vi "SCMP FITS Writer.vi"(5 "Andor":T1={"Handle"=0, "Pixel Encoding"="", "AOI Width"=0, "AOI Height"=0, "AOI Stride"=0, "Row Readout Time"=0.0, "Frame Readout Time"=0.0, "Interframe Time"=0.0, "Semaphore"=refnum, "SerialNumber"="", "Camera Model"="", "Controller ID"="", "Firmware Version"="", "Shutter"="Global", "BDiv"=1, "Time at Synch"=timestamp(3029526000.379448 s since 1904-01-01), "Idx"=0, "PreAmp"="", "Binning"=enum."1x1", "PixelReadoutRate"="", "Exposure (s)"=0.05, "Image Bytes"=0, "Image Pixels"=0, "SpuriousNoiseFilter"=FALSE, "Overlap"=FALSE, "CycleMode"=""} {"Exposure (s)" format="%^.3g"; "Time at Synch" format="%<%H:%M:%S>T"; "Interframe Time" format="%#_3g"; "Frame Readout Time" format="%_3g"; "Row Readout Time" format="%_3g"}, 7 "FITS Cluster":T4={"Wavelength (nm)"=530.15, "Exposure (s)"=0.05, "Tuning Delay (ms)"=1000.0, "Beam Type (-1/1)"=1.0, "Tuning Voltages"=[1.111, 2.222, 3.333, 4.444], "Observer"="observer", "Light Shapping Diffuser"=enum."In Beam", "Comment"="", "Data Type"=9, "Mod Cycles"=0, "SCD Calibration Optics"=enum."1 - Polarizer @0, I+Q", "SCD Emission Line Filter"=enum."1-557.6nm", "Cookbook"="", "COMP-S Calibration Wheel"=enum."Dark", "COMP-S Andover Filter Wheel"=enum."530.3nm/HWB 0.34nm (Fe XIV)", "FOV Rotation (deg)"=66.0, "Objective Lens Position (mm)"=0.0, "Occulter size"=0.0, "Time End"=timestamp(3382374145.421875 s since 1904-01-01), "Acc Exposure (s)"=0.0, "Time Stamp Array"=[], "Camera Serial Number"=[], "Camera Temp"=[], "Camera PI (mm)"=[], "Time Start"=timestamp(3382374145.421875 s since 1904-01-01), "Peripherals"={"ILX controler"=FALSE, "Zone temperatures"=FALSE, "Andor"=FALSE, "Andor 2"=FALSE, "PI Stages"=FALSE, "AISAS mechanisms"=FALSE, "AISAS Mech.lvclass"=refnum, "Zone temp ref"=variant, "FWs"=FALSE}, "FITS paths"=[], "Cameras"=enum."Andor", "load preset cbk"=FALSE, "periodic check count"=0} {"Camera PI (mm)" format="%_3g"; "Acc Exposure (s)" format="%^.3g"; "Occulter size" format="%.2f"; "Objective Lens Position (mm)" min=70.0 max=152.0 format="%.2f"; "FOV Rotation (deg)" format="%.1f"; "Data Type" items=["LIVE", "DARK", "FLAT", "CALI", "OBSE", "ABSO", "AURE", "TARG", "OBJE", "HOLE", "OREX", "THRO", "CHIP"]; "Exposure (s)" format="%^.3g"; "Wavelength (nm)" format="%_6g"}, 8 "error in":errorcluster, 10 "Image Vector":u32[](array[numeric]), 11 "Wavelength (0..n)":i32) -> (0 "error out":errorcluster, 3 "Current FITS Path":path)   [LabVIEW 2014]
doc: "Use this template to build a VI to use as a subVI."
uses:
  Controls/SCD - FITS Cluster.ctl
  AISAS/Mech/AISAS Mech.lvclass
  AISAS/Controls/Diffuser.ctl
  Controls/SCD - Calibration Optics Filter Wheel.ctl
  Controls/SCD - EDT - Emission Line Filter Wheel.ctl
  Controls/CoMP-S Controls/Polarization Optics Filter Wheel.ctl
  Controls/CoMP-S Controls/Emission Line Filter Wheel.ctl
  AISAS/Controls/focus.ctl
  Controls/peripherals.ctl
  Controls/Cameras select.ctl
  Camera/Andor Neo Info.ctl
  Controls/beaning.ctl
panel:
  out "FITS Path static":path=path "G:/SCD Data/Level-0/20160930/20160930T203514.fits"
  out "1st Extension Header":string="XTENSION=                        'IMAGE' /                                      BITPIX  =                             32 / BITS PER PIXEL                       NAXIS   =                              3 / NUMBER OF AXES (2)                   NAXIS1  =                           2560 / XDIM (PIXELS)                        NAXIS2  =                           2160 / YDIM (PIXELS)                        NAXIS3  =                              4 / 4 POLARIZATION STATES                GCOUNT  =                              1 /                                      TIME_OBS=                   '203202.348' / TIME OF OBSERVATION (UTC)            DATE_END=                                / DATE OF OBSERVATION END (UTC)        EXPOSURE=                       0.020000 / EXPOSURE TIME (MILLISEC)             PCOUNT  =                              0 /                                      BZERO   =                             0. / 32768.                               BSCALE  =                             1. / 1                                    MODC    =                              3 / NUMBER OF IMAGES AT EACH STATE       WAVELENG=                         656.20 / WAVELENGTH OF OBS (NM)               COMMENT                                                                         COMMENT                                                                         COMMENT                                                                         COMMENT                                                                         COMMENT                                                                         COMMENT                                                                         COMMENT                                                                         COMMENT                                                                         COMMENT                                                                         COMMENT                                                                         COMMENT                                                                         COMMENT                                                                         COMMENT                                                                         COMMENT                                                                         COMMENT                                                                         COMMENT                                                                         COMMENT                                                                         COMMENT                                                                         COMMENT                                                                         COMMENT                                                                         COMMENT                                                                         COMMENT                                                                         COMMENT                                                                         COMMENT                                                                         COMMENT                                                                         COMMENT                                                                         COMMENT                                                                         COMMENT                                                                         COMMENT                                                                         COMMENT                                                                         COMMENT                                                                         COMMENT                                                                         COMMENT                                                                         COMMENT                                                                         COMMENT                                                                         COMMENT                                                                         COMMENT                                                                         COMMENT                                                                         COMMENT                                                                         COMMENT                                                                         COMMENT                                                                         COMMENT                                                                         COMMENT                                                                         COMMENT                                                                         COMMENT                                                                         COMMENT                                                                         COMMENT                                                                         COMMENT                                                                         COMMENT                                                                         COMMENT                                                                         COMMENT                                                                         COMMENT                                                                         COMMENT                                                                         COMMENT                                                                         COMMENT                                                                         COMMENT                                                                         COMMENT                                                                         COMMENT                                                                         COMMENT                                                                         COMMENT                                                                         COMMENT                                                                         COMMENT                                                                         COMMENT                                                                         COMMENT                                                                         COMMENT                                                                         COMMENT                                                                         COMMENT                                                                         COMMENT                                                                         COMMENT                                                                         COMMENT                                                                         COMMENT                                                                         COMMENT                                                                         COMMENT                                                                         COMMENT                                                                         COMMENT                                                                         COMMENT                                                                         COMMENT                                                                         COMMENT                                                                         COMMENT                                                                         COMMENT                                                                         COMMENT                                                                         COMMENT                                                                         COMMENT                                                                         COMMENT                                                                         COMMENT                                                                         COMMENT                                                                         COMMENT                                                                         COMMENT                                                                         COMMENT                                                                         COMMENT                                                                         COMMENT                                                                         COMMENT                                                                         COMMENT                                                                         COMMENT                                                                         COMMENT                                                                         COMMENT                                                                         COMMENT                                                                         COMMENT                                                                         COMMENT                                                                         COMMENT                                                                         COMMENT                                                                         COMMENT                                                                         COMMENT                                                                         COMMENT                                                                         COMMENT                                                                         COMMENT                                                                         COMMENT                                                                         COMMENT                                                                         COMMENT                                                                         COMMENT                                                                         COMMENT                                                                         COMMENT                                                                         COMMENT                                                                         COMMENT                                                                         COMMENT                                                                         COMMENT                                                                         COMMENT                                                                         COMMENT                                                                         COMMENT                                                                         COMMENT                                                                         COMMENT                                                                         COMMENT                                                                         COMMENT                                                                         COMMENT                                                                         COMMENT                                                                         COMMENT                                                                         COMMENT                                                                         COMMENT                                                                         COMMENT                                                                         COMMENT                                                                         COMMENT                                                                         COMMENT                                                                         COMMENT                                                                         COMMENT                                                                         COMMENT                                                                         COMMENT                                                                         COMMENT                                                                         COMMENT                                                                         COMMENT                                                                         COMMENT                                                                         COMMENT                                                                         COMMENT                                                                         COMMENT                                                                         COMMENT                                                                         COMMENT                                                                         COMMENT                                                                         COMMENT                                                                         COMMENT                                                                         COMMENT                                                                         COMMENT                                                                         COMMENT                                                                         COMMENT                                                                         COMMENT                                                                         COMMENT                                                                         COMMENT                                                                         COMMENT                                                                         COMMENT                                                                         COMMENT                                                                         COMMENT                                                                         COMMENT                                                                         COMMENT                                                                         COMMENT                                                                         COMMENT                                                                         COMMENT                                                                         COMMENT                                                                         COMMENT                                                                         COMMENT                                                                         COMMENT                                                                         COMMENT                                                                         COMMENT                                                                         COMMENT                                                                         COMMENT                                                                         COMMENT                                                                         COMMENT                                                                         COMMENT                                                                         COMMENT                                                                         COMMENT                                                                         COMMENT                                                                         COMMENT                                                                         COMMENT                                                                         COMMENT                                                                         COMMENT                                                                         COMMENT                                                                         COMMENT                                                                         COMMENT                                                                         COMMENT                                                                         COMMENT                                                                         COMMENT                                                                         COMMENT                                                                         COMMENT                                                                         COMMENT                                                                         COMMENT                                                                         COMMENT                                                                         COMMENT                                                                         COMMENT                                                                         COMMENT                                                                         COMMENT                                                                         COMMENT                                                                         COMMENT                                                                         COMMENT                                                                         COMMENT                                                                         COMMENT                                                                         COMMENT                                                                         COMMENT                                                                         COMMENT                                                                         COMMENT                                                                         COMMENT                                                                         COMMENT                                                                         COMMENT                                                                         COMMENT                                                                         COMMENT                                                                         COMMENT                                                                         COMMENT                                                                         COMMENT                                                                         COMMENT                                                                         COMMENT                                                                         COMMENT                                                                         COMMENT                                                                         COMMENT                                                                         COMMENT                                                                         COMMENT                                                                         COMMENT                                                                         COMMENT                                                                         COMMENT                                                                         COMMENT                                                                         COMMENT                                                                         COMMENT                                                                         COMMENT                                                                         COMMENT                                                                         COMMENT                                                                         COMMENT                                                                         COMMENT                                                                         COMMENT                                                                         COMMENT                                                                         COMMENT                                                                         COMMENT                                                                         COMMENT                                                                         COMMENT                                                                         COMMENT                                                                         COMMENT                                                                         COMMENT                                                                         COMMENT                                                                         COMMENT                                                                         COMMENT                                                                         COMMENT                                                                         COMMENT                                                                         COMMENT                                                                         COMMENT                                                                         COMMENT                                                                         COMMENT                                                                         COMMENT                                                                         COMMENT                                                                         COMMENT                                                                         COMMENT                                                                         COMMENT                                                                         COMMENT                                                                         COMMENT                                                                         COMMENT                                                                         COMMENT                                                                         COMMENT                                                                         COMMENT                                                                         COMMENT                                                                         COMMENT                                                                         COMMENT                                                                         COMMENT                                                                         COMMENT                                                                         COMMENT                                                                         COMMENT                                                                         COMMENT                                                                         COMMENT                                                                         COMMENT                                                                         COMMENT                                                                         END                                                                             "
  out "Primary Header":string="SIMPLE  =                              T / CONFORMS TO FITS STANDARD            BITPIX  =                             32 / BITS PER PIXEL                       NAXIS   =                              0 / DATA DIMENSIONS IN FITS FILE         NAXIS1  =                           2560 / XDIM (PIXELS)                        NAXIS2  =                           2160 / YDIM (PIXELS)                        NAXIS3  =                              4 / 4 POLARIZATION STATES                NAXIS4  =                              1 / 1 CAMERA                             EXTEND  =                              T / EXTENSIONS POSSIBLE                  OBSERVER=                       'Sewell' / NAME OF OBSERVER                     TELESCOP=                   '20CM ZEISS' / NAME OF TELESCOPE                    LOCATION=            'LOMNICKY PEAK OBS' / LOCATION OF TELESCOPE                INSTRUME=                          'SCD' / NAME OF INSTRUMENT                   BZERO   =                             0. /  ADU OFFSET                          FOCUS   =                     -22.000000 / CAMERA-STAGE POSITION (MM)           ROTPOS  =                            0.0 / ROTATIONAL POSITION (DEG)            DIFFUSER=                      'IN BEAM' / 0=IN BEAM, 1=OUT OF BEAM             FW-WVLNG=                        '656.4' / PRE-FILTER CENTER WAVELENGTH (NM)    FW-CALIB=                         'Dark' / CAL-WHEEL POSITION                   CAM-SN1 =                    'SCC-02209' / CAMERA SERIAL NUMBER                 CAM-TEMP=                     -19.610000 / FOCAL PLANE TEMP (C)                 TUNEDLAY=                            200 / LCVR RELAXATION DELAY (mS)           DATE_OBS=                    '9/30/2016' / DATE OF OBSERVATION START (UTC)      TIME_OBS=                   '203202.348' / TIME OF OBSERVATION (UTC)            EXPOSURE=                       0.020000 / EXPOSURE TIME (S)                    MODC    =                              3 / NUMBER OF IMAGES AT EACH STATE       NLC-1   =                          1.607 / TUNING VOLTAGE-1                     NLC-2   =                          2.450 / TUNING VOLTAGE-2                     NLC-3   =                          2.243 / TUNING VOLTAGE-3                     NLC-4   =                          2.518 / TUNING VOLTAGE-4                     NLC-5   =                          2.067 / TUNING VOLTAGE-5                     BEAM    =                              1 / BEAM (0=ON BAND OR 1=CONTINUUM)      WAVELENG=                         656.20 / WAVELENGTH OF OBS (NM)               COMMHEAD=               'Extension Test' / OBSERVER COMMENT                     COOKBOOK=              scotts-tester.cbk / COOKBOOK  LOADED                     DATATYPE=                           DARK / IMAGE TYPE                           ORIGIN  =                        'AISAS' / SCIENTIFIC GROUP                     COMMENT                                                                         COMMENT                                                                         COMMENT                                                                         COMMENT                                                                         COMMENT                                                                         COMMENT                                                                         COMMENT                                                                         COMMENT                                                                         COMMENT                                                                         COMMENT                                                                         COMMENT                                                                         COMMENT                                                                         COMMENT                                                                         COMMENT                                                                         COMMENT                                                                         COMMENT                                                                         COMMENT                                                                         COMMENT                                                                         COMMENT                                                                         COMMENT                                                                         COMMENT                                                                         COMMENT                                                                         COMMENT                                                                         COMMENT                                                                         COMMENT                                                                         COMMENT                                                                         COMMENT                                                                         COMMENT                                                                         COMMENT                                                                         COMMENT                                                                         COMMENT                                                                         COMMENT                                                                         COMMENT                                                                         COMMENT                                                                         COMMENT                                                                         COMMENT                                                                         COMMENT                                                                         COMMENT                                                                         COMMENT                                                                         COMMENT                                                                         COMMENT                                                                         COMMENT                                                                         COMMENT                                                                         COMMENT                                                                         COMMENT                                                                         COMMENT                                                                         COMMENT                                                                         COMMENT                                                                         COMMENT                                                                         COMMENT                                                                         COMMENT                                                                         COMMENT                                                                         COMMENT                                                                         COMMENT                                                                         COMMENT                                                                         COMMENT                                                                         COMMENT                                                                         COMMENT                                                                         COMMENT                                                                         COMMENT                                                                         COMMENT                                                                         COMMENT                                                                         COMMENT                                                                         COMMENT                                                                         COMMENT                                                                         COMMENT                                                                         COMMENT                                                                         COMMENT                                                                         COMMENT                                                                         COMMENT                                                                         COMMENT                                                                         COMMENT                                                                         COMMENT                                                                         COMMENT                                                                         COMMENT                                                                         COMMENT                                                                         COMMENT                                                                         COMMENT                                                                         COMMENT                                                                         COMMENT                                                                         COMMENT                                                                         COMMENT                                                                         COMMENT                                                                         COMMENT                                                                         COMMENT                                                                         COMMENT                                                                         COMMENT                                                                         COMMENT                                                                         COMMENT                                                                         COMMENT                                                                         COMMENT                                                                         COMMENT                                                                         COMMENT                                                                         COMMENT                                                                         COMMENT                                                                         COMMENT                                                                         COMMENT                                                                         COMMENT                                                                         COMMENT                                                                         COMMENT                                                                         COMMENT                                                                         COMMENT                                                                         COMMENT                                                                         COMMENT                                                                         COMMENT                                                                         COMMENT                                                                         COMMENT                                                                         COMMENT                                                                         COMMENT                                                                         COMMENT                                                                         COMMENT                                                                         COMMENT                                                                         COMMENT                                                                         COMMENT                                                                         COMMENT                                                                         COMMENT                                                                         COMMENT                                                                         COMMENT                                                                         COMMENT                                                                         COMMENT                                                                         COMMENT                                                                         COMMENT                                                                         COMMENT                                                                         COMMENT                                                                         COMMENT                                                                         COMMENT                                                                         COMMENT                                                                         COMMENT                                                                         COMMENT                                                                         COMMENT                                                                         COMMENT                                                                         COMMENT                                                                         COMMENT                                                                         COMMENT                                                                         COMMENT                                                                         COMMENT                                                                         COMMENT                                                                         COMMENT                                                                         COMMENT                                                                         COMMENT                                                                         COMMENT                                                                         COMMENT                                                                         COMMENT                                                                         COMMENT                                                                         COMMENT                                                                         COMMENT                                                                         COMMENT                                                                         COMMENT                                                                         COMMENT                                                                         COMMENT                                                                         COMMENT                                                                         COMMENT                                                                         COMMENT                                                                         COMMENT                                                                         COMMENT                                                                         COMMENT                                                                         COMMENT                                                                         COMMENT                                                                         COMMENT                                                                         COMMENT                                                                         COMMENT                                                                         COMMENT                                                                         COMMENT                                                                         COMMENT                                                                         COMMENT                                                                         COMMENT                                                                         COMMENT                                                                         COMMENT                                                                         COMMENT                                                                         COMMENT                                                                         COMMENT                                                                         COMMENT                                                                         COMMENT                                                                         COMMENT                                                                         COMMENT                                                                         COMMENT                                                                         COMMENT                                                                         COMMENT                                                                         COMMENT                                                                         COMMENT                                                                         COMMENT                                                                         COMMENT                                                                         COMMENT                                                                         COMMENT                                                                         COMMENT                                                                         COMMENT                                                                         COMMENT                                                                         COMMENT                                                                         COMMENT                                                                         COMMENT                                                                         COMMENT                                                                         COMMENT                                                                         COMMENT                                                                         COMMENT                                                                         COMMENT                                                                         COMMENT                                                                         COMMENT                                                                         COMMENT                                                                         COMMENT                                                                         COMMENT                                                                         COMMENT                                                                         COMMENT                                                                         COMMENT                                                                         COMMENT                                                                         COMMENT                                                                         COMMENT                                                                         COMMENT                                                                         COMMENT                                                                         COMMENT                                                                         COMMENT                                                                         COMMENT                                                                         COMMENT                                                                         COMMENT                                                                         COMMENT                                                                         COMMENT                                                                         COMMENT                                                                         COMMENT                                                                         COMMENT                                                                         COMMENT                                                                         COMMENT                                                                         COMMENT                                                                         COMMENT                                                                         COMMENT                                                                         COMMENT                                                                         COMMENT                                                                         COMMENT                                                                         COMMENT                                                                         COMMENT                                                                         COMMENT                                                                         COMMENT                                                                         COMMENT                                                                         COMMENT                                                                         COMMENT                                                                         COMMENT                                                                         COMMENT                                                                         COMMENT                                                                         COMMENT                                                                         COMMENT                                                                         COMMENT                                                                         COMMENT                                                                         COMMENT                                                                         COMMENT                                                                         COMMENT                                                                         COMMENT                                                                         COMMENT                                                                         COMMENT                                                                         COMMENT                                                                         COMMENT                                                                         COMMENT                                                                         COMMENT                                                                         COMMENT                                                                         END                                                                             "
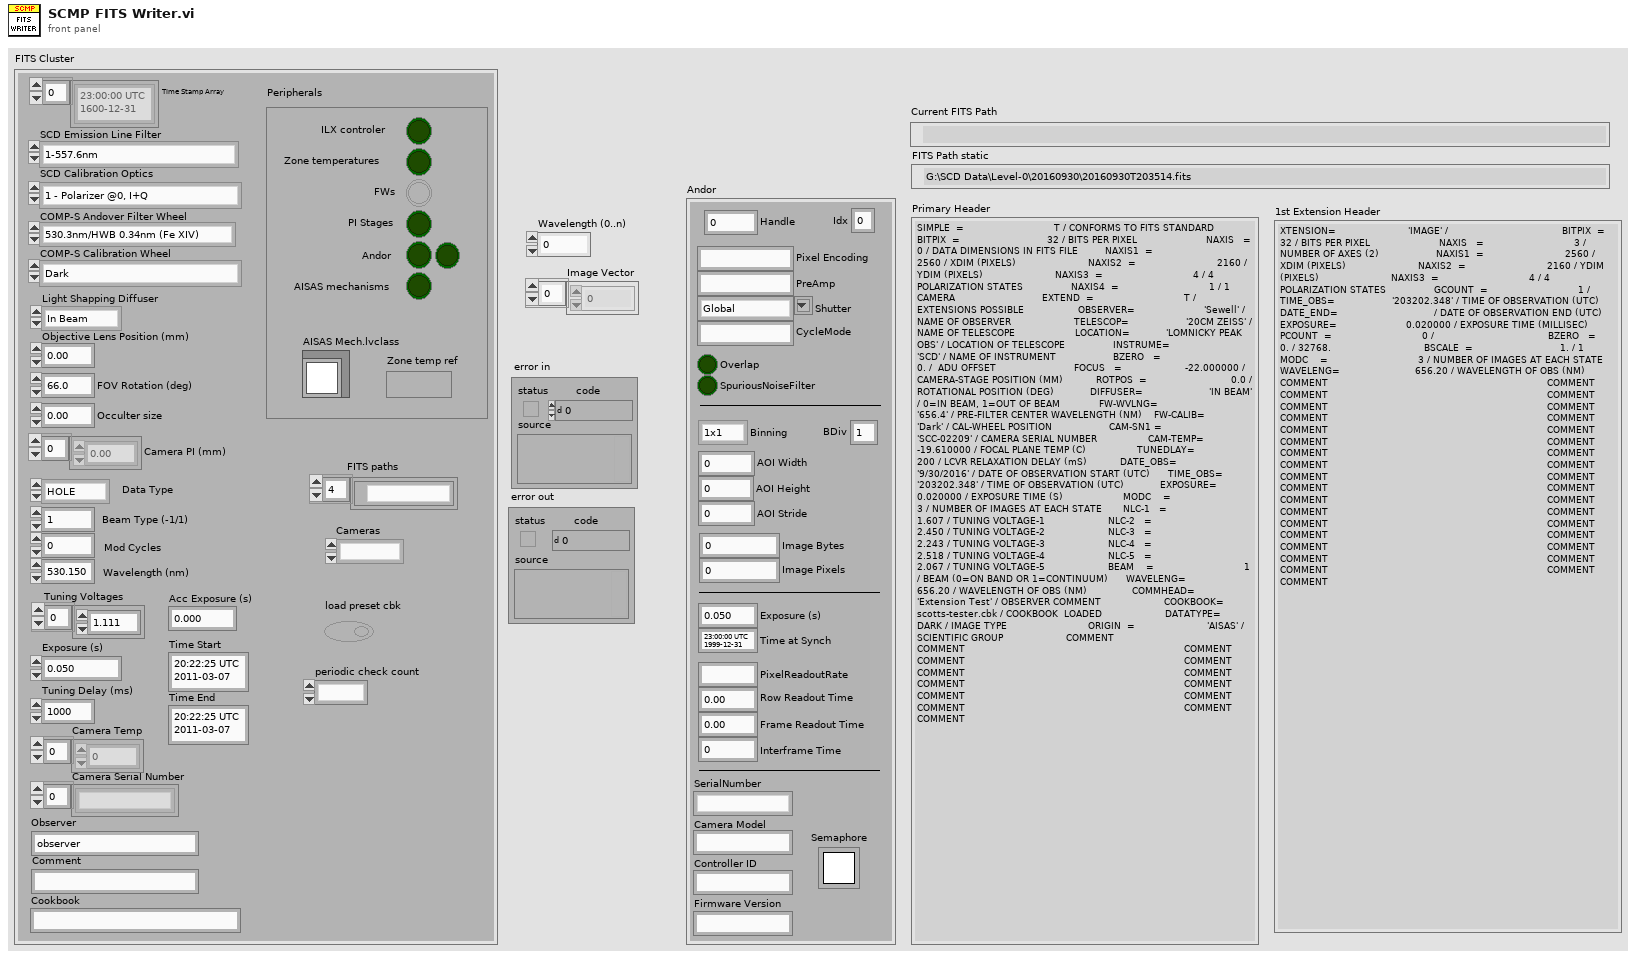
[diagram p1: front panel]
types:
  T1 = typedef "Andor Neo Info.ctl" = cluster{"Handle":i32, "Pixel Encoding":string, "AOI Width":i32, "AOI Height":i32, "AOI Stride":i32, "Row Readout Time":dbl, "Frame Readout Time":dbl, "Interframe Time":dbl, "Semaphore":T2, "SerialNumber":string, "Camera Model":string, "Controller ID":string, "Firmware Version":string, "Shutter":string, "BDiv":u8, "Time at Synch":timestamp, "Idx":i32, "PreAmp":string, "Binning":T3, "PixelReadoutRate":string, "Exposure (s)":dbl, "Image Bytes":i64, "Image Pixels":i64, "SpuriousNoiseFilter":bool, "Overlap":bool, "CycleMode":string}
  T2 = typedef "Semaphore RefNum" = refnum<k1>
  T3 = typedef "beaning.ctl" = enum16{"1x1", "2x2", "3x3", "4x4", "8x8"}
  T4 = typedef "SCD - FITS Cluster.ctl" = cluster{"Wavelength (nm)":dbl, "Exposure (s)":dbl, "Tuning Delay (ms)":dbl, "Beam Type (-1/1)":dbl, "Tuning Voltages":dbl[], "Observer":string, "Light Shapping Diffuser":T5, "Comment":string, "Data Type":u16, "Mod Cycles":u16, "SCD Calibration Optics":T6, "SCD Emission Line Filter":T7, "Cookbook":string, "COMP-S Calibration Wheel":T8, "COMP-S Andover Filter Wheel":T9, "FOV Rotation (deg)":dbl, "Objective Lens Position (mm)":T10, "Occulter size":dbl, "Time End":timestamp, "Acc Exposure (s)":dbl, "Time Stamp Array":timestamp[], "Camera Serial Number":string[], "Camera Temp":dbl[], "Camera PI (mm)":dbl[], "Time Start":timestamp, "Peripherals":T11, "FITS paths":path[], "Cameras":T12, "load preset cbk":bool, "periodic check count":i32}
  T5 = typedef "Diffuser.ctl" = enum16{"Out of Beam", "In Beam"}
  T6 = typedef "SCD - Calibration Optics Filter Wheel.ctl" = enum16{"1 - Polarizer @0, I+Q", "2 - Polarizer @90, I-Q", "3 - Polarizer @45, I+U", "4 - Polarizer @135, I-U", "5 - Polarizer @0, Retarder @45, I+V", "6 - Polarizer @0, Retarder @135, I-V", "7 - Dark", "8 - Clear", "9 - N/A"}
  T7 = typedef "SCD - EDT - Emission Line Filter Wheel.ctl" = enum16{"1-557.6nm", "2-587.6nm", "3-589.6nm", "4-630.2nm", "5-656.4nm", "6-849.8nm", "7-854.2nm", "8-866.2nm", "9-1083.0nm"}
  T8 = typedef "Polarization Optics Filter Wheel.ctl" = enum16{"Dark", "Clear", "Exchange Lens", "Polarizer @0, I+Q", "Polarizer @90, I-Q", "Polarizer @45, I+U", "Polarizer @135, I-U", "Polarizer @0, Retarder @45, I+V", "Polarizer @0, Retarder @135, I-V"}
  T9 = typedef "Emission Line Filter Wheel.ctl" = enum16{"530.3nm/HWB 0.34nm (Fe XIV)", "587.6nm/HBW 0.44nm (He I D3)", "637.5nm/HBW 0.53nm (Fe X)", "656.3nm/HBW 0.57nm (H-Alpha)", "789.2nm/HBW 0.85nm (Fe XI)", "854.2nm/HBW 1.01nm (Ca I)", "1074.7nm/HBW 2.34nm (Fe XIII)", "1079.8nm/HBW 1.64nm (Fe XIII)", "1083.0nm/HBW 1.66nm (He I)"}
  T10 = typedef "focus.ctl" = dbl
  T11 = typedef "peripherals.ctl" = cluster{"ILX controler":bool, "Zone temperatures":bool, "Andor":bool, "Andor 2":bool, "PI Stages":bool, "AISAS mechanisms":bool, "AISAS Mech.lvclass":refnum<class "AISAS Mech.lvclass">, "Zone temp ref":variant, "FWs":bool}
  T12 = typedef "Cameras select.ctl" = enum16{"Andor", "GDR"}
  T13 = typedef "Fits info.ctl" = cluster{"File name":string, "Date":string}
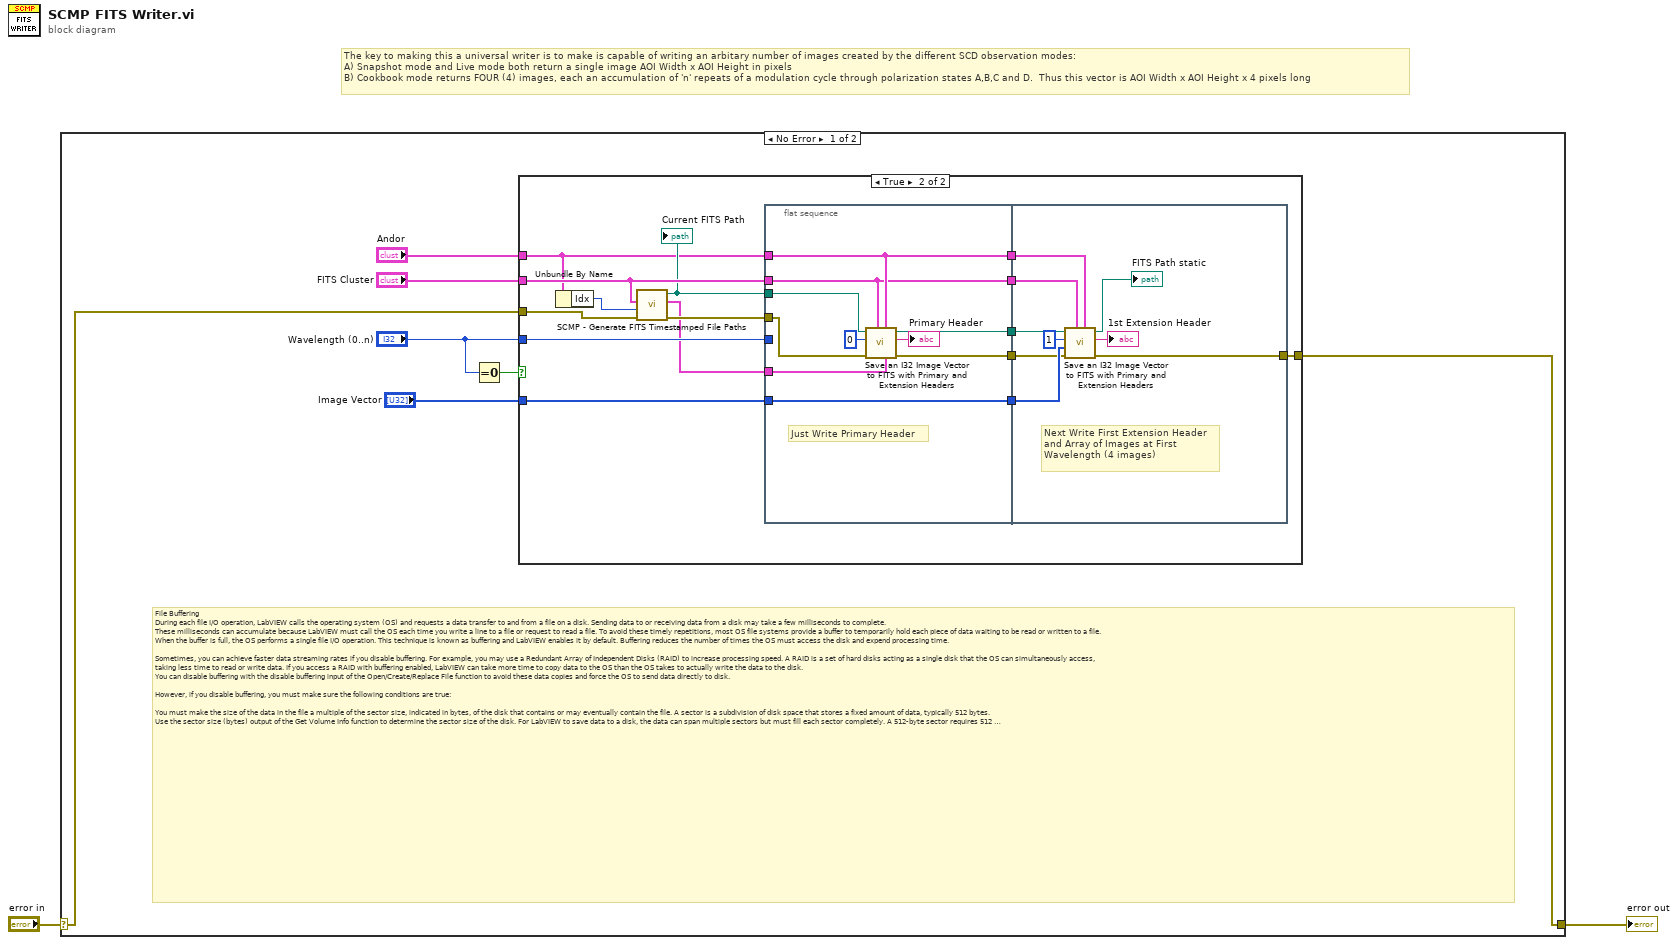
[diagram p0: block diagram]
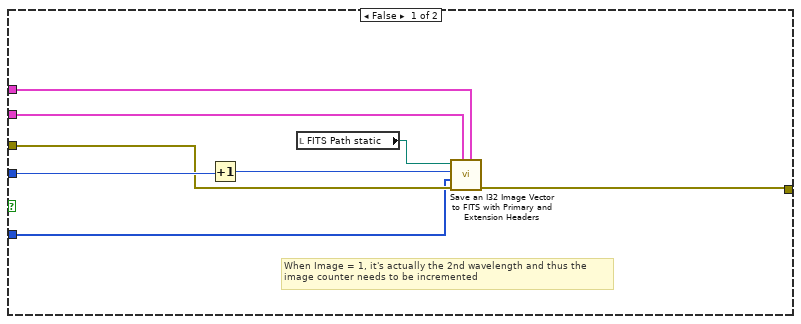
[diagram p2: hidden frame]
diagram:
  # "The key to making this a universal writer is to make is capable of writing an arbitary number of images created by the different SCD observation modes:\nA) Snapshot mode and Live mode both return a single image AOI Width x AOI Height in pixels\nB) Cookbook mode returns FOUR (4) images, each an accumulation of 'n' repeats of a modulation cycle through polarization states A,B,C and D.  Thus this vector is AOI Width x AOI Height x 4 pixels long"
  n1 = case shown="No Error" "error in" {
    selector: "error in" -> [w7 w52]
    tunnel: [w6 w52] -> w1
    frame No Error {
      # "File Buffering\nDuring each file I/O operation, LabVIEW calls the operating system (OS) and requests a data transfer to and from a file on a disk. Sending data to or receiving data from a disk may take a few milliseconds to complete. \nThese milliseconds can accumulate because LabVIEW must call the OS each time you write a line to a file or request to read a file. To avoid these timely repetitions, most OS file systems provide a buffer to temporarily hold each piece of data waiting to be read or written to a file. \nWhen the buffer is full, the OS performs a single file I/O operation. This technique is known as buffering and LabVIEW enables it by default. Buffering reduces the number of times the OS must access the disk and expend processing time. \n\nSometimes, you can achieve faster data streaming rates if you disable buffering. For example, you may use a Redundant Array of Independent Disks (RAID) to increase processing speed. A RAID is a set of hard disks acting as a single disk that the OS can simultaneously access, \ntaking less time to read or write data. If you access a RAID with buffering enabled, LabVIEW can take more time to copy data to the OS than the OS takes to actually write the data to the disk. \nYou can disable buffering with the disable buffering input of the Open/Create/Replace File function to avoid these data copies and force the OS to send data directly to disk.\n\nHowever, if you disable buffering, you must make sure the following conditions are true:\n\nYou must make the size of the data in the file a multiple of the sector size, indicated in bytes, of the disk that contains or may eventually contain the file. A sector is a subdivision of disk space that stores a fixed amount of data, typically 512 bytes. \nUse the sector size (bytes) output of the Get Volume Info function to determine the sector size of the disk. For LabVIEW to save data to a disk, the data can span multiple sectors but must fill each sector completely. A 512-byte sector requires 512 bytes of data. \nIf the data is not a multiple of the sector size, you must pad the data with filler data and delete the filler data before LabVIEW reads back the file. \nThe data in the file must be aligned to a multiple of the alignment the disk requires. LabVIEW aligns the data, and you cannot change that alignment. If the data does not meet the alignment requirement, LabVIEW returns an error and you must enable buffering and reopen the file."
      n2 = Equal To 0?(x="Wavelength (0..n)") -> (x = 0?=w4:bool)
      n3 = case shown="True" w4 {
        tunnel: "Wavelength (0..n)" -> [w17 w31]
        tunnel: "Andor" -> [w12 w19]
        tunnel: "FITS Cluster" -> [w13 w22]
        tunnel: "Image Vector" -> [w11 w28]
        tunnel: w7 -> [w15 w23]
        tunnel: [w14 w26] -> w6
        frame False {
          # "When Image = 1, it's actually the 2nd wavelength and thus the\nimage counter needs to be incremented"
          n4 = Increment(x=w17) -> (x+1=w16:i32)
          n5 = local read "FITS Path static"() -> (w10:path)
          n6 = call "Save an I32 Image Vector to FITS with Primary and Extension Headers.vi"("Andor"=w12, "SCD FITS Cluster"=w13, "error in"=w15, "Image Data"=w11, "Image #"=w16, "FITS File Path"=w10) -> ("error out"=w14:errorcluster)  [unwired: 3 in, 2 out]
        }
        frame True {
          n7 = Unbundle By Name(w19) -> ("Idx"=w18:i32)
          n8 = call "SCMP - Generate FITS Timestamped File Paths.vi"("error in"=w23, "Camera Idx"=w18, "FITS Header"=w22) -> ("error out"=w24:errorcluster, "FITS info"=w21:T13, "FITS File Path"=w20:path)  [unwired: 6 in]
          "Current FITS Path" <- w20
          n9 = flat-sequence {
            tunnel: w31 -> [_]
            tunnel: w19 -> [w42]
            tunnel: w22 -> [w35]
            tunnel: [w42] -> w32
            tunnel: w20 -> [w33]
            tunnel: [w41] -> w30
            tunnel: [w39] -> w29
            tunnel: w28 -> [w39]
            tunnel: w24 -> [w38]
            tunnel: [w37] -> w27
            tunnel: [w35] -> w25
            tunnel: w21 -> [w34]
            tunnel: w32 -> [w51]
            tunnel: w30 -> [w50]
            tunnel: w29 -> [w48]
            tunnel: w27 -> [w47]
            tunnel: [w46] -> w26
            tunnel: w25 -> [w43]
            frame #0 {
              # "Just Write Primary Header"
              n10 = call "Save an I32 Image Vector to FITS with Primary and Extension Headers.vi"("FITS info"=w34, "Andor"=w42, "SCD FITS Cluster"=w35, "error in"=w38, "Image #"=0, "FITS File Path"=w33) -> ("error out"=w37:errorcluster, "23040 Byte Header"=→"Primary Header":string, "FITS Path Out"=w41:path)  [unwired: 3 in]
            }
            frame #1 {
              # "Next Write First Extension Header\nand Array of Images at First\nWavelength (4 images)"
              n11 = call "Save an I32 Image Vector to FITS with Primary and Extension Headers.vi"("Andor"=w51, "SCD FITS Cluster"=w43, "error in"=w47, "Image Data"=w48, "Image #"=1, "FITS File Path"=w50) -> ("error out"=w46:errorcluster, "23040 Byte Header"=→"1st Extension Header":string, "FITS Path Out"=→"FITS Path static":path)  [unwired: 3 in]
            }
          }
        }
      }
    }
    frame Error {
    }
  }
  "error out" <- w1
